vi "Sigmoid.vi"(1 "Z matrix":T1) -> (0 "Sigmoid":T1)   [LabVIEW 2016]
uses:
  <vilib>/Analysis/Matrix/Datatypes/RealMatrix.ctl
  <vilib>/Analysis/Matrix/Numeric/Add/Add (Elementwise) - R,RM.vi
  <vilib>/Analysis/Matrix/NI_Matrix.lvlib
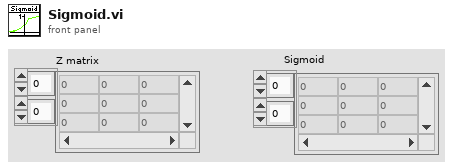
[diagram p1: front panel]
types:
  T1 = typedef "NI_Matrix.lvlib/RealMatrix.ctl" = dbl[][]
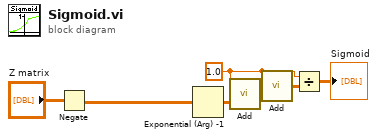
[diagram p0: block diagram]
diagram:
  w3 = 1.0
  n1 = Negate(x="Z matrix") -> (-x=w6:T1)
  n2 = Exponential (Arg) -1(1:w6) -> (0:w7:T1)
  n3 = call-poly <vilib>:"Add.vi"("Real Matrix A"=w7, "Real Scalar c"=w3) -> ("c + A"=w4:T1)
  n4 = call-poly <vilib>:"Add.vi"("Real Matrix A"=w4, "Real Scalar c"=w3) -> ("c + A"=w5:T1)
  n5 = Divide(x=w3, y=w5) -> (x/y=→"Sigmoid":T1)
